vi "WRITE HEADER CSV.vi"(10 "Array":string[](array[string]), 11 "file path":path) -> (3 "Byte Stream File out":refnum<file>)   [LabVIEW 2016]
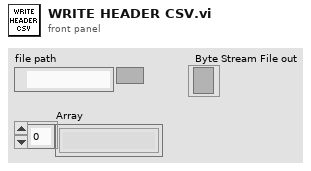
[diagram p1: front panel]
types:
  T1 = enum16{"open", "replace", "create", "open or create", "replace or create", "replace or create with confirmation"}
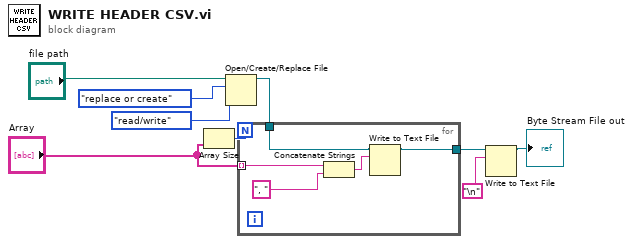
[diagram p0: block diagram]
diagram:
  n1 = Array Size(array="Array") -> (size(s)=w4:i32)
  n2 = Open/Create/Replace File(file path (use dialog)="file path", operation (0:open)=T1."replace or create", access (0:read/write)=enum16{"read/write", "read-only", "write-only"}."read/write") -> (refnum out=w6:refnum<file>)  [unwired: 3 in, 2 out]
  n3 = for {
    N: w4 -> [_]
    tunnel: w6 -> [w12]
    tunnel: "Array" -> [w14] mode=indexing
    tunnel: [w11] -> w7
    n4 = Concatenate Strings(w14, ", ") -> (w13:string)
    n5 = Write to Text File(file (use dialog)=w12, text=w13) -> (refnum out=w11:refnum<file>)  [unwired: 2 in, 2 out]
  }
  n6 = Write to Text File(file (use dialog)=w7, text="\n") -> (refnum out=→"Byte Stream File out":refnum<file>)  [unwired: 2 in, 2 out]
